vi "Process Motor Current.vi"(10 "bHighCurrentOK":bool, 11 "IHighCurrent":fxp<+/-,19,15>) -> (1 "bIMotorCalculated":bool, 3 "IMotor":dbl)   [LabVIEW 2015]
uses:
  Global Data.vi
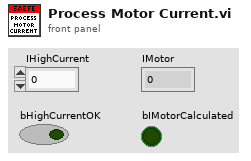
[diagram p1: front panel]
types:
  T1 = typedef "MC Current.ctl" = cluster{"IMCPhaseA":dbl, "IMCPhaseB":dbl, "IMCPhaseC":dbl, "IMCBatteryCalc":dbl}
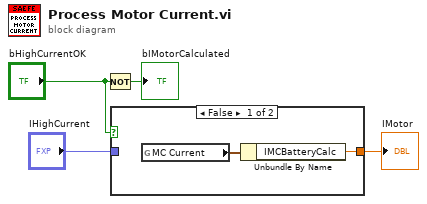
[diagram p0: block diagram]
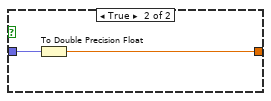
[diagram p2: hidden frame]
diagram:
  n1 = Not(x="bHighCurrentOK") -> (.not. x?=→"bIMotorCalculated":bool)
  n2 = case shown="False" "bHighCurrentOK" {
    tunnel: "IHighCurrent" -> [_ w8]
    tunnel: [w5 w7] -> w4
    frame False {
      n3 = global read "Global Data.vi" "MC Current"() -> (w6:T1)
      n4 = Unbundle By Name(w6) -> ("IMCBatteryCalc"=w5:dbl)
    }
    frame True {
      n5 = To Double Precision Float(number=w8) -> (double precision float=w7:dbl)
    }
  }
  "IMotor" <- w4
